vi "FABR-Read Data.vi"(0 "Data files":path[](array[path]), 11 "error in (no error)":errorcluster) -> (4 "Analysis":T1, 15 "error out":errorcluster)   [LabVIEW 2020]
uses:
  Typedefs/FABR-Analysis State.ctl
  Threshold Estimation VIs/ABR3-Threshold Estimation Result.ctl
panel:
  # "Freq X Level X Time"
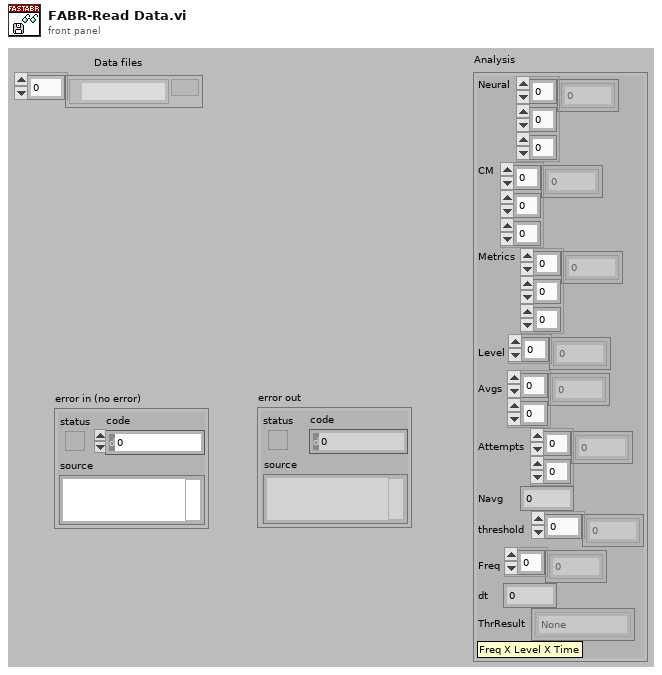
[diagram p1: front panel]
types:
  T1 = typedef "FABR-Analysis State.ctl" = cluster{"Neural":dbl[][][], "CM":dbl[][][], "Metrics":dbl[][][], "Level":dbl[], "Avgs":i32[][], "Attempts":i32[][], "Navg":i32, "threshold":dbl[], "Freq":dbl[], "dt":dbl, "ThrResult":T2[]}
  T2 = typedef "ABR3-Threshold Estimation Result.ctl" = enum16{"None", "Power", "Sigmoid", "Power (noisy)", "Suprathreshold", "Invalid"}
  T3 = typedef "FABR-Header.ctl" = cluster{"Path":path, "Date":string, "Chamber":string, "CFTS":string, "StartTime":string, "EndTime":string, "Frequency (kHz)":dbl, "Levels":string, "Avgs":string, "Tries":string, "ThrResult":T2, "Threshold":dbl, "Notes":string}
  T4 = typedef "FABR-Parameters.ctl" = cluster{"Format":i32, "Stimulus":T5, "Sequence":T6, "Response":T8, "Reject":dbl}
  T5 = typedef "FABR-Stimulus.ctl" = cluster{"Destination":string, "Rep rate (/sec)":dbl, "Alternate Polarity":bool, "Duration (ms)":dbl, "Ramp (ms)":dbl, "Fs (Hz)":dbl, "Frame size (s)":dbl}
  T6 = typedef "FABR-Sequence.ctl" = cluster{"Freq":cluster{"Expression":string, "Skip":i32}, "Level":cluster{"Start (dB)":i32, "Stop (dB)":i32, "Step (dB)":i32}, "Order":T7}
  T7 = typedef "FABR-Order.ctl" = enum16{"Interleaved"}
  T8 = typedef "FABR-Response.ctl" = cluster{"Gain":dbl, "Averages":i32, "Window (ms)":sgl, "Fs (Hz)":dbl, "Save raw":bool}
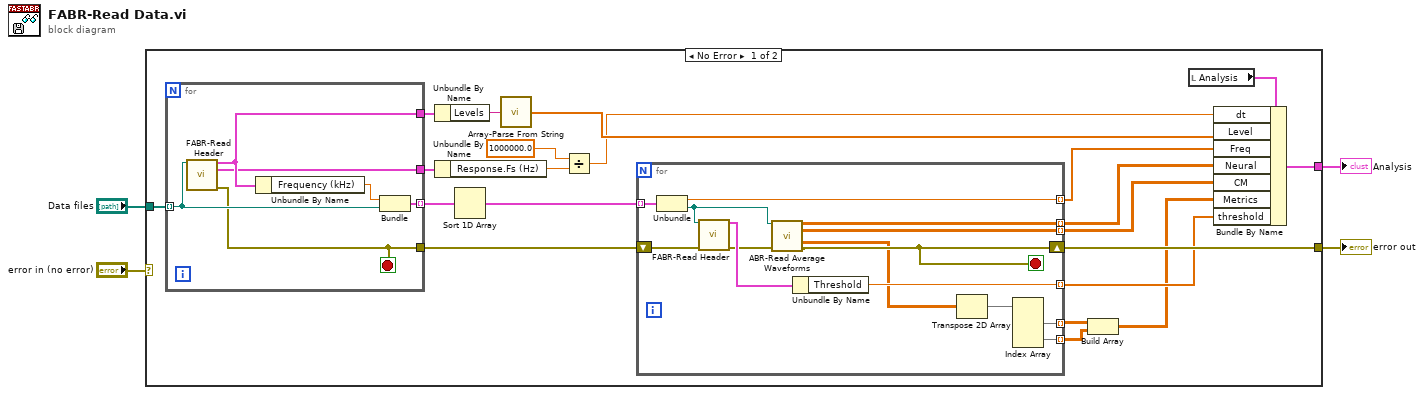
[diagram p0: block diagram]
diagram:
  n1 = case shown="No Error" "error in (no error)" {
    selector: "error in (no error)" -> [_ w46]
    tunnel: [w17 w46] -> w3
    tunnel: "Data files" -> [w24 _]
    tunnel: [w25 _] -> w1
    frame No Error {
      n2 = for {
        tunnel: w24 -> [w45] mode=indexing
        tunnel: [w44] -> w23 mode=indexing
        tunnel: [w41] -> w20
        tunnel: [w42] -> w18
        tunnel: [w40] -> w11
        stop <- w42 stop-if-true
        n3 = call "FABR-Read Header.vi"("Path"=w45) -> ("Header"=w41:T3, "Params"=w40:T4, "error out"=w42:errorcluster)  [unwired: 12 in]
        n4 = Unbundle By Name(w41) -> ("Frequency (kHz)"=w43:dbl)
        n5 = Bundle("Frequency (kHz)"=w43, "Path"=w45) -> (w44:cluster{"Frequency (kHz)":dbl, "Path":path})  [unwired: 1 in]
      }
      n6 = Unbundle By Name(w20) -> ("Levels"=w13:string)
      n7 = Unbundle By Name(w11) -> ("Response.Fs (Hz)"=w10:dbl)
      n8 = Sort 1D Array(array=w23) -> (sorted array=w22:cluster{"Frequency (kHz)":dbl, "Path":path}[])
      n9 = call "Array-Parse From String.vi"("String"=w13) -> ("Array"=w12:dbl[])  [unwired: 13 in, 1 out]
      n10 = Divide(x=1000000.0, y=w10) -> (x/y=w8:dbl)
      n11 = for {
        tunnel: w22 -> [w39] mode=indexing
        tunnel: [w38] -> w19 mode=indexing
        shift-right: [w30] -> w17
        shift-left: w18 -> [w37]
        tunnel: [w32] -> w16 mode=indexing
        tunnel: [w31] -> w15 mode=indexing
        tunnel: [w35] -> w14 mode=indexing
        tunnel: [w27] -> w7 mode=indexing
        tunnel: [w26] -> w6 mode=indexing
        stop <- w30 stop-if-true
        n12 = Unbundle(w39) -> ("Frequency (kHz)"=w38:dbl, "Path"=w34:path)
        n13 = call "FABR-Read Header.vi"("Path"=w34, "error in (no error)"=w37) -> ("Header"=w36:T3, "error out"=w33:errorcluster)  [unwired: 11 in, 1 out]
        n14 = call "ABR-Read Average Waveforms.vi"("Path"=w34, "error in"=w33) -> ("Neural"=w32:dbl[][], "CM"=w31:dbl[][], "Metrics"=w29:dbl[][], "error out"=w30:errorcluster)  [unwired: 10 in]
        n15 = Unbundle By Name(w36) -> ("Threshold"=w35:dbl)
        n16 = Transpose 2D Array(2D array=w29) -> (transposed array=w28:dbl[][])
        n17 = Index Array(array=w28) -> (element #1=w27:dbl[], element #2=w26:dbl[])  [unwired: 4 in]
      }
      n18 = Build Array(w7, w6) -> (w5:dbl[][][])
      n19 = local read "Analysis"() -> (w21:T1)
      n20 = Bundle By Name(cluster=w21, "dt"=w8, "Level"=w12, "Freq"=w19, "Neural"=w16, "CM"=w15, "Metrics"=w5, "threshold"=w14) -> (w25:T1)
    }
    frame Error {
    }
  }
  "error out" <- w3
  "Analysis" <- w1
